vi "Update run counter file.vi"(8 "error in (no error)":errorcluster, 11 "run counter path":path) -> (0 "error out":errorcluster, 2 "Run ID":i32, 3 "Process cancelled":bool)   [LabVIEW 2016]
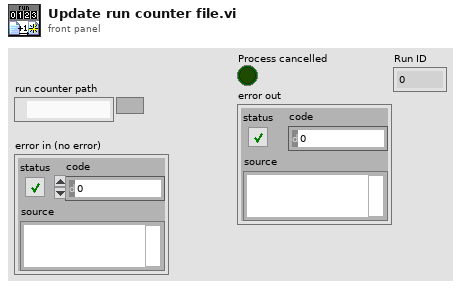
[diagram p1: front panel]
types:
  T1 = enum16{"open", "replace", "create", "open or create", "replace or create", "replace or create with confirmation"}
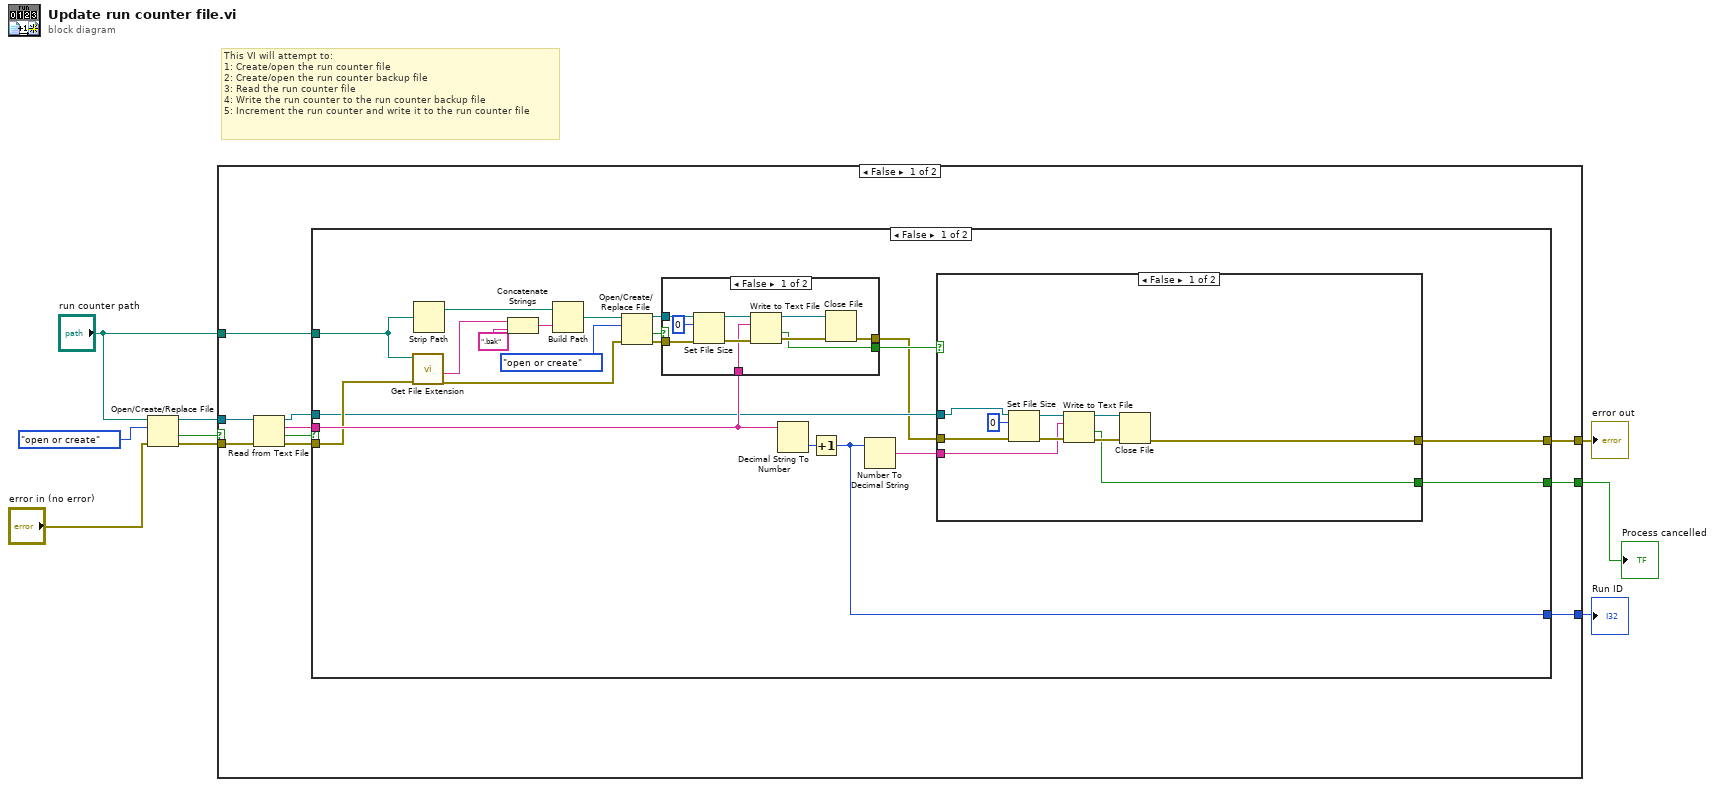
[diagram p0: block diagram]
diagram:
  # "This VI will attempt to:\n1: Create/open the run counter file \n2: Create/open the run counter backup file\n3: Read the run counter file\n4: Write the run counter to the run counter backup file\n5: Increment the run counter and write it to the run counter file"
  n1 = Open/Create/Replace File(file path (use dialog)="run counter path", error in="error in (no error)", operation (0:open)=T1."open or create") -> (refnum out=w9:refnum<file>, cancelled=w4:bool, error out=w8:errorcluster)  [unwired: 3 in]
  n2 = case shown="False" w4 {
    selector: w4 -> [_ w68]
    tunnel: w9 -> [w19 _]
    tunnel: w8 -> [w18 w67]
    tunnel: "run counter path" -> [w16 _]
    tunnel: [w12 w68] -> w3
    tunnel: [w11 w67] -> w2
    tunnel: [w10 _] -> w1
    frame False {
      n3 = Read from Text File(file (use dialog)=w19, error in=w18) -> (refnum out=w13:refnum<file>, text=w17:string, cancelled=w14:bool, error out=w15:errorcluster)  [unwired: 2 in]
      n4 = case shown="False" w14 {
        selector: w14 -> [_ w66]
        tunnel: w17 -> [w31 _]
        tunnel: w16 -> [w30 _]
        tunnel: w15 -> [w29 w65]
        tunnel: w13 -> [w25 _]
        tunnel: [w22 w66] -> w12
        tunnel: [w21 w65] -> w11
        tunnel: [w20 _] -> w10
        frame False {
          n5 = call <vilib>:"Get File Extension.vi"("error in (no error)"=w29, "file"=w30) -> ("error out"=w28:errorcluster, "filename without extension"=w38:string)  [unwired: 5 in, 3 out]
          n6 = Strip Path(path=w30) -> (stripped path=w37:path)  [unwired: 1 out]
          n7 = Concatenate Strings(w38, ".bak") -> (w36:string)
          n8 = Build Path(base path=w37, name or relative path=w36) -> (appended path=w35:path)
          n9 = Open/Create/Replace File(file path (use dialog)=w35, error in=w28, operation (0:open)=T1."open or create") -> (refnum out=w32:refnum<file>, cancelled=w27:bool, error out=w33:errorcluster)  [unwired: 3 in]
          n10 = case shown="False" w27 {
            selector: w27 -> [_ w63]
            tunnel: w33 -> [w62 w64]
            tunnel: w32 -> [w61 _]
            tunnel: w31 -> [w57 _]
            tunnel: [w54 w63] -> w26
            tunnel: [w53 w64] -> w24
            frame False {
              n11 = Set File Size(4:w62, 6:i64 0 ("size (in bytes)"), 7:w61) -> (0:w59:errorcluster, 3:w58:refnum<file>)
              n12 = Write to Text File(file (use dialog)=w58, text=w57, error in=w59) -> (refnum out=w55:refnum<file>, cancelled=w54:bool, error out=w56:errorcluster)  [unwired: 1 in]
              n13 = Close File(refnum=w55, error in=w56) -> (error out=w53:errorcluster)  [unwired: 1 out]
            }
            frame True {
            }
          }
          n14 = Decimal String To Number(string=w31) -> (number=w40:i32)  [unwired: 2 in, 1 out]
          n15 = Increment(x=w40) -> (x+1=w20:i32)
          n16 = Number To Decimal String(number=w20) -> (decimal integer string=w23:string)  [unwired: 1 in]
          n17 = case shown="False" w26 {
            selector: w26 -> [_ w52]
            tunnel: w25 -> [w49 _]
            tunnel: w24 -> [w48 w51]
            tunnel: w23 -> [w45 _]
            tunnel: [w42 w52] -> w22
            tunnel: [w41 w51] -> w21
            frame False {
              n18 = Set File Size(4:w48, 6:i64 0 ("size (in bytes)"), 7:w49) -> (0:w47:errorcluster, 3:w46:refnum<file>)
              n19 = Write to Text File(file (use dialog)=w46, text=w45, error in=w47) -> (refnum out=w43:refnum<file>, cancelled=w42:bool, error out=w44:errorcluster)  [unwired: 1 in]
              n20 = Close File(refnum=w43, error in=w44) -> (error out=w41:errorcluster)  [unwired: 1 out]
            }
            frame True {
            }
          }
        }
        frame True {
        }
      }
    }
    frame True {
    }
  }
  "Process cancelled" <- w3
  "error out" <- w2
  "Run ID" <- w1
